vi "Read Tasks names.vi"(8 "error in (no error)":errorcluster caption="entrée d'erreur (pas d'erreur)", 11 "DAQmxTaskContainer en entrée":refnum<class "DAQmxTaskContainer.lvclass">) -> (0 "error out":errorcluster caption="sortie d'erreur", 2 "Tasks names":string[](array[string]), 3 "DAQmxTaskContainer en sortie":refnum<class "DAQmxTaskContainer.lvclass">)   [LabVIEW 2015, in "DAQmxTaskContainer.lvclass"]
uses:
  DAQmxTaskContainer.lvclass
  DAQmxTaskContainer.lvclass/DAQmxTaskContainer.ctl
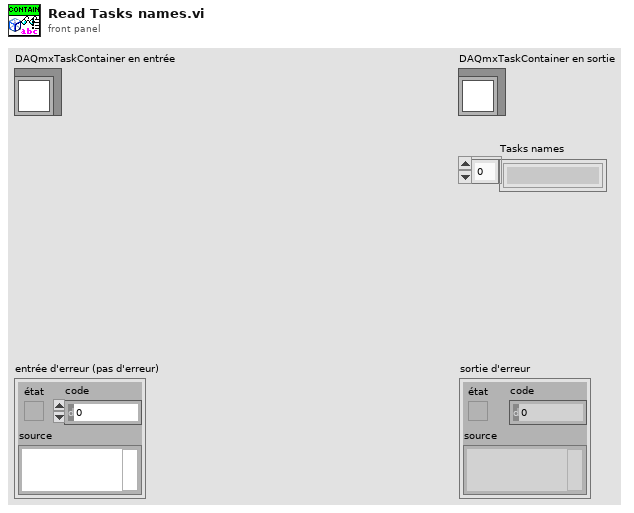
[diagram p1: front panel]
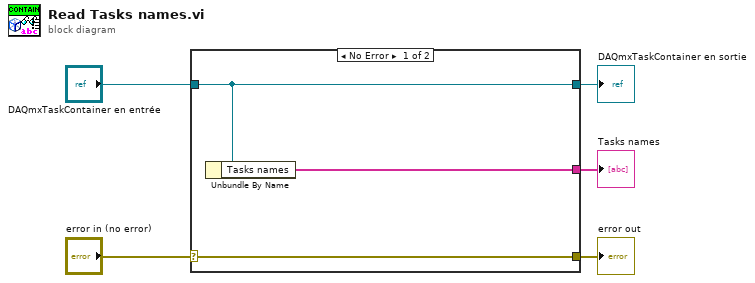
[diagram p0: block diagram]
diagram:
  n1 = case shown="No Error" "error in (no error)" {
    selector: "error in (no error)" -> [w8 w9]
    tunnel: [w8 w9] -> w4
    tunnel: [w7 w10] -> w2
    tunnel: "DAQmxTaskContainer en entrée" -> [w7 w10]
    tunnel: [w6 _] -> w1
    frame No Error {
      n2 = Unbundle By Name(w7) -> ("Tasks names"=w6:string[])
    }
    frame Error {
    }
  }
  "error out" <- w4
  "DAQmxTaskContainer en sortie" <- w2
  "Tasks names" <- w1
